vi "new-CSAC-GPS.vi"() -> ()   [LabVIEW 2024]
uses:
  <vilib>/Instr/_visa.llb/VISA Configure Serial Port (Instr).vi
  <vilib>/regexp/Match Regular Expression.xnode
panel:
  in  "single file name":string="24NESMA_NODE_GPS"
  in  "log path":string="D:\\24NESMA\\GPS log\\"
  in  "Boolean 2":bool
  in  "Boolean":bool=TRUE
  out "date/time string":string
  out "before match 4":string
  out "before match 3":string
  out "before match 2":string
  out "before match":string
  out "read buffer":string
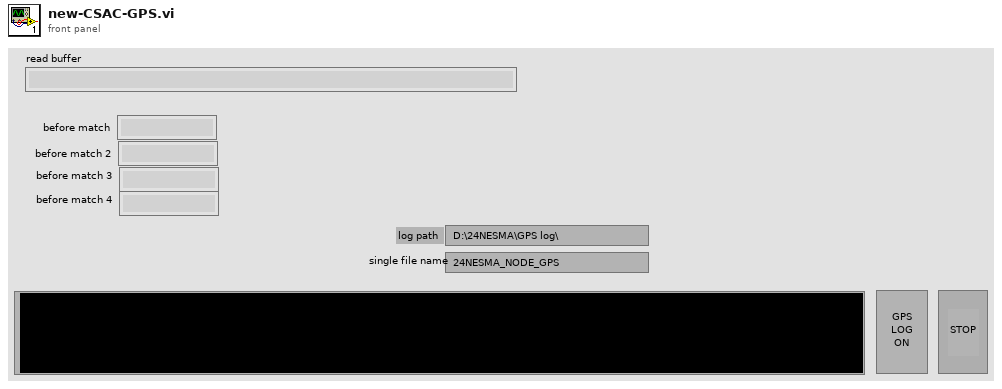
[diagram p1: front panel]
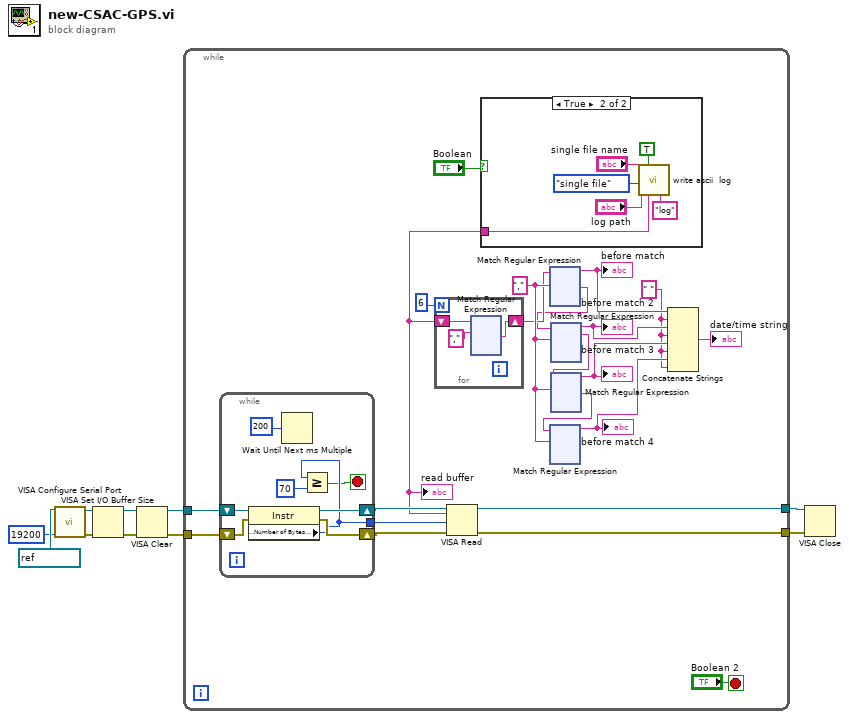
[diagram p0: block diagram]
diagram:
  n1 = call-poly "VISA Configure Serial Port"("VISA resource name"=refnum<visa-resource-name> "COM3", "baud rate (9600)"=u32 19200) -> ("VISA resource name out"=w7:refnum<visa-resource-name>, "error out"=w8:errorcluster)  [unwired: 12 in]
  n2 = VISA Set I/O Buffer Size(VISA resource name=w7, error in (no error)=w8) -> (VISA resource name out=w4:refnum<visa-resource-name>, error out=w3:errorcluster)  [unwired: 2 in]
  n3 = VISA Clear(VISA resource name=w4, error in (no error)=w3) -> (VISA resource name out=w2:refnum<visa-resource-name>, error out=w1:errorcluster)
  n4 = while {
    tunnel: w2 -> [w25]
    tunnel: w1 -> [w32]
    tunnel: [w29] -> w6
    tunnel: [w28] -> w5
    stop <- "Boolean 2" stop-if-true
    w13 = " " ("string")
    w23 = "," ("search string/char (-)")
    n5 = while {
      tunnel: [w630] -> w27
      shift-right: [w632] -> w31
      shift-left: w32 -> [w633]
      shift-right: [w631] -> w30
      shift-left: w25 -> [w628]
      stop <- w627 stop-if-true
      n6 = property class="Instr"(reference=w628, error in=w633) -> (reference out=w631:refnum<visa-resource-name>, error out=w632:errorcluster, "Serial Settings:Number of Bytes at Serial Port"=w630:u32)
      n7 = Wait Until Next ms Multiple(millisecond multiple=u32 200) -> ()  [unwired: 1 out]
      n8 = Greater Or Equal?(x=w630, y=u32 70) -> (x >= y?=w627:bool)
    }
    n9 = VISA Read(VISA resource name=w30, byte count=w27, error in (no error)=w31) -> (VISA resource name out=w28:refnum<visa-resource-name>, read buffer=w11:string, error out=w29:errorcluster)  [unwired: 1 out]
    "read buffer" <- w11
    n10 = for {
      N: 6 -> [_]
      shift-right: [w507] -> w22
      shift-left: w11 -> [w509]
      n11 = xnode "Match Regular Expression"("input string"=w509, "regular expression"="," ("search string/char (-)")) -> ("after match"=w507:string)  [unwired: 4 in, 4 out]
    }
    n12 = case shown="True" "Boolean" {
      tunnel: w11 -> [_ w36]
      frame False {
      }
      frame True {
        n13 = call "write ascii  log.vi"("single file name"="single file name", "logging on/off"=TRUE, "log path"="log path", "hourly(0)/daily(1)"=enum16{"hourly", "daily", "single file"}."single file", "ASCII data"=w36, "extension"="log") -> ()  [unwired: 9 in, 1 out]
      }
    }
    n14 = xnode "Match Regular Expression"("input string"=w22, "regular expression"=w23) -> ("before match"=w17:string, "after match"=w21:string)  [unwired: 4 in, 3 out]
    "before match" <- w17
    n15 = xnode "Match Regular Expression"("input string"=w21, "regular expression"=w23) -> ("before match"=w16:string, "after match"=w20:string)  [unwired: 4 in, 3 out]
    "before match 2" <- w16
    n16 = xnode "Match Regular Expression"("input string"=w20, "regular expression"=w23) -> ("before match"=w15:string, "after match"=w19:string)  [unwired: 4 in, 3 out]
    "before match 3" <- w15
    n17 = xnode "Match Regular Expression"("input string"=w19, "regular expression"=w23) -> ("before match"=w14:string)  [unwired: 4 in, 4 out]
    "before match 4" <- w14
    n18 = Concatenate Strings(w17, w13, w16, w13, w15, w13, w14, w13) -> (→"date/time string":string)
  }
  n19 = VISA Close(VISA resource name=w5, error in (no error)=w6) -> ()  [unwired: 1 out]
